vi "01-guageonly.vi"() -> ()   [LabVIEW 2026]
uses:
  <vilib>/Utility/error.llb/Trim Whitespace One-Sided.vi
panel:
  in  "stop":bool
  out "Gauge":dbl(knob) scale=0.0..100.0
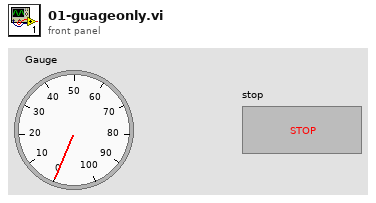
[diagram p1: front panel]
types:
  T1 = enum16{"Standard", "Buffered", "CRLF", "Immediate"}
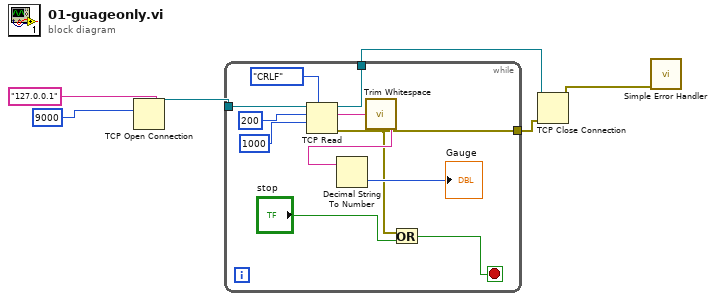
[diagram p0: block diagram]
diagram:
  n1 = TCP Open Connection(address="127.0.0.1", remote port or service name=9000) -> (connection ID=w4:refnum<k5>)  [unwired: 3 in, 1 out]
  n2 = while {
    tunnel: w4 -> [w17]
    tunnel: [w10] -> w2
    tunnel: [w9] -> w1
    stop <- w7 stop-if-true
    n3 = TCP Read(connection ID=w17, bytes to read=200, 7:T1."CRLF" ("mode (standard)"), 9:1000) -> (connection ID out=w10:refnum<k5>, data out=w13:string, error out=w9:errorcluster)  [unwired: 1 in]
    n4 = call <vilib>:"Trim Whitespace.vi"("string"=w13) -> ("trimmed string"=w12:string)  [unwired: 1 in]
    n5 = Decimal String To Number(string=w12) -> (number=→"Gauge":i32)  [unwired: 2 in, 1 out]
    n6 = Or(x=w9, y="stop") -> (x .or. y?=w7:bool)
  }
  n7 = TCP Close Connection(connection ID=w2, error in (no error)=w1) -> (error out=w3:errorcluster)  [unwired: 1 in, 1 out]
  n8 = call <vilib>:"Simple Error Handler.vi"("error in (no error)"=w3) -> ()  [unwired: 4 in, 5 out]
